vi "readAndWriteSerial_7102.vi"(8 "error in (no error)":errorcluster {"code" format="%.0x"}, 10 "Write Buffer (\"\")":string, 11 "instrument handle":refnum<k15>) -> (0 "error out":errorcluster {"code" format="%.0x"}, 2 "Read Buffer":string, 3 "instrument handle out":refnum<k15>)   [LabVIEW 2015, in "SerialCommunication.lvlib"]
uses:
  SerialCommunication.lvlib
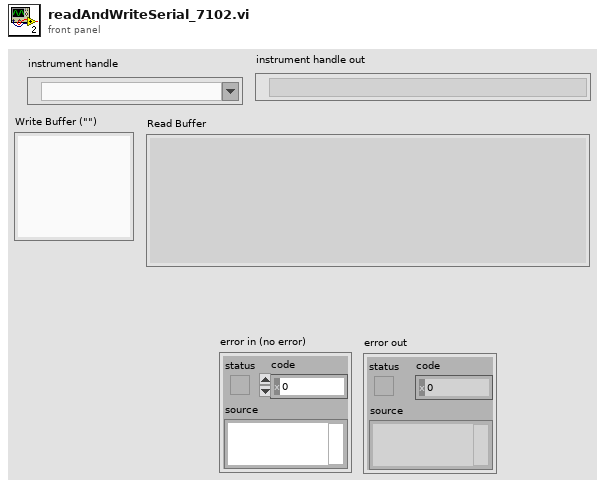
[diagram p1: front panel]
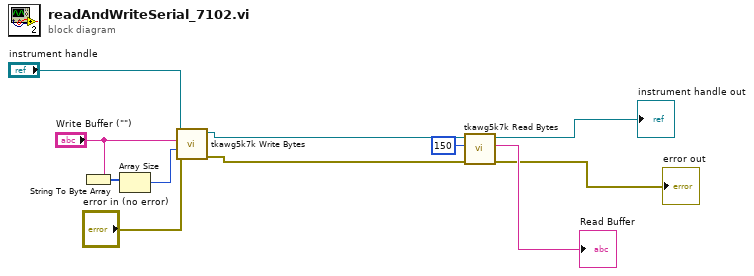
[diagram p0: block diagram]
diagram:
  n1 = String To Byte Array(string="Write Buffer (\"\")") -> (unsigned byte array=w7:u8[])
  n2 = Array Size(array=w7) -> (size(s)=w6:i32)
  n3 = call <instrlib>:"tkawg5k7k Write Bytes.vi"("error in (no error)"="error in (no error)", "Number of Bytes to Write"=w6, "Write Buffer (\"\")"="Write Buffer (\"\")", "instrument handle"="instrument handle") -> ("error out"=w10:errorcluster, "instrument handle out"=w11:refnum<k15>)  [unwired: 5 in, 1 out]
  n4 = call <instrlib>:"tkawg5k7k Read Bytes.vi"("error in (no error)"=w10, "Number of Bytes to Read"=i64 150, "instrument handle"=w11) -> ("error out"=→"error out":errorcluster, "Read Buffer"=→"Read Buffer":string, "instrument handle out"=→"instrument handle out":refnum<k15>)  [unwired: 5 in, 1 out]
